vi "(TestVI)Overflow.vi"(7 "Init":bool, 11 "Data in":u16[][](array[numeric])) -> (3 "Data out":i32[][](array[numeric]))   [LabVIEW 2020]
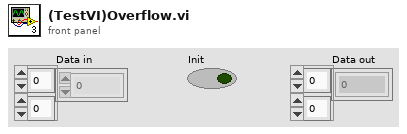
[diagram p1: front panel]
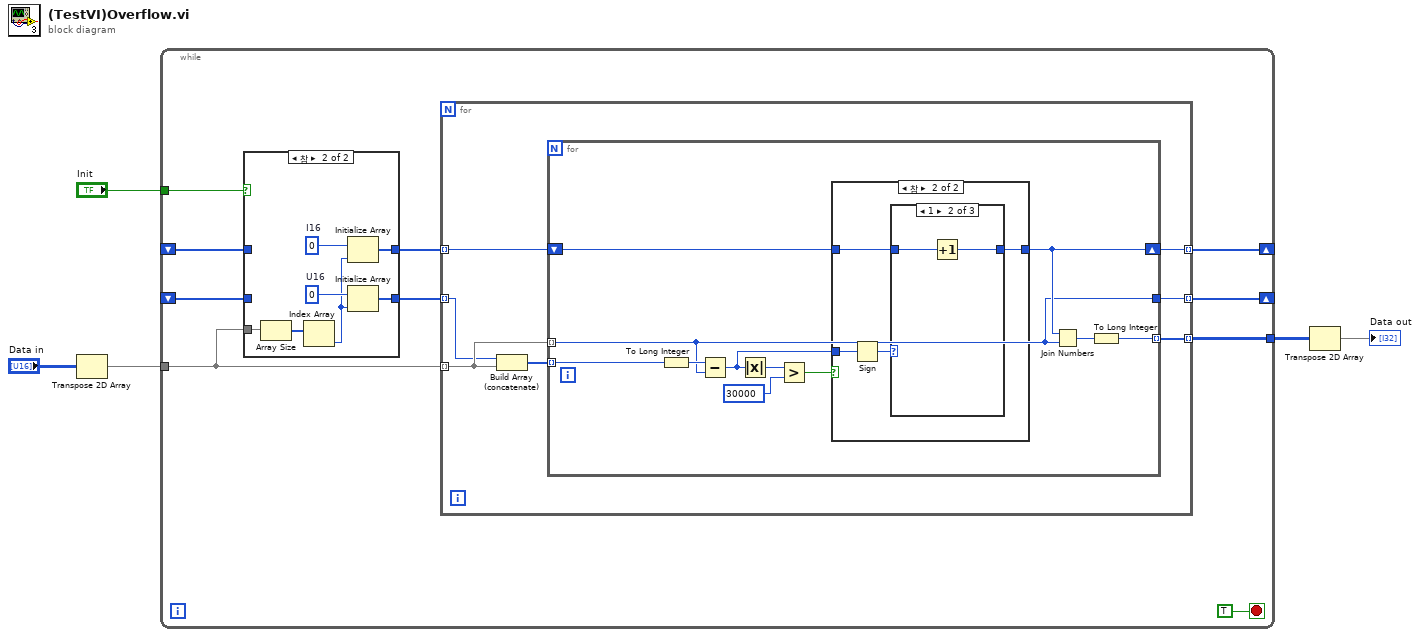
[diagram p0: block diagram]
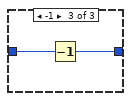
[diagram p5: hidden frame]
diagram:
  n1 = Transpose 2D Array(2D array="Data in") -> (transposed array=w4:u16[][])
  n2 = while {
    tunnel: w4 -> [w10]
    tunnel: [w15] -> w3
    shift-right: [w13] -> _
    shift-left: _ -> [w6]
    shift-right: [w12] -> _
    shift-left: _ -> [w9]
    tunnel: "Init" -> [w11]
    stop <- TRUE stop-if-true
    n3 = case shown="참" w11 {
      tunnel: w10 -> [_ w24]
      tunnel: w9 -> [w17 _]
      tunnel: [w17 w21] -> w8
      tunnel: [w16 w18] -> w7
      tunnel: w6 -> [w16 _]
      frame False {
      }
      frame True {
        w20 = u16 0  # U16
        w23 = i16 0  # I16
        n4 = Array Size(array=w24) -> (size(s)=w22:i32[])
        n5 = Index Array(array=w22) -> (element=w19:i32)  [unwired: 1 in]
        n6 = Initialize Array(w23, w19) -> (w21:i16[])
        n7 = Initialize Array(w20, w19) -> (w18:u16[])
      }
    }
    n8 = for {
      tunnel: w10 -> [w31] mode=indexing
      tunnel: w8 -> [w30] mode=indexing
      tunnel: [w29] -> w15 mode=indexing
      tunnel: [w28] -> w13 mode=indexing
      tunnel: w7 -> [w25] mode=indexing
      tunnel: [w26] -> w12 mode=indexing
      n9 = Build Array (concatenate)(w25, w31) -> (w27:u16[])
      n10 = for {
        tunnel: w27 -> [w32] mode=indexing
        tunnel: w31 -> [w33] mode=indexing
        tunnel: [w36] -> w29 mode=indexing
        shift-right: [w34] -> w26
        shift-left: w30 -> [w39]
        tunnel: [w33] -> w28
        n11 = To Long Integer(number=w32) -> (32bit integer=w38:i32)
        n12 = Subtract(x=w38, y=w33) -> (x-y=w40:i32)
        n13 = Absolute Value(x=w40) -> (abs(x)=w42:i32)
        n14 = Greater?(x=w42, y=30000) -> (0:w35:bool)
        n15 = case shown="참" w35 {
          tunnel: w40 -> [_ w47]
          tunnel: w39 -> [w43 w45]
          tunnel: [w43 w44] -> w34
          frame False {
          }
          frame True {
            n16 = Sign(1:w47) -> (0:w46:i32)
            n17 = case shown="1" w46 {
              tunnel: w45 -> [w48 w50 w52]
              tunnel: [w48 w49 w51] -> w44
              frame 0, Default {
              }
              frame 1 {
                n18 = Increment(x=w50) -> (x+1=w49:i16)
              }
              frame -1 {
                n19 = Decrement(x=w52) -> (x-1=w51:i16)
              }
            }
          }
        }
        n20 = Join Numbers(hi=w34, lo=w33) -> ((hi.lo)=w37:u32)
        n21 = To Long Integer(number=w37) -> (32bit integer=w36:i32)
      }
    }
  }
  n22 = Transpose 2D Array(2D array=w3) -> (transposed array=→"Data out":i32[][])
